vi "BuildPacket.vi"(1 "Data":u8[](array[numeric]), 2 "TxID":u32) -> (0 "MsgTX 2":T1)   [LabVIEW 2010]
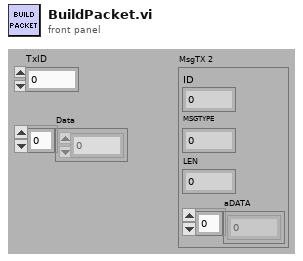
[diagram p1: front panel]
types:
  T1 = cluster{"ID":u32, "MSGTYPE":u8, "LEN":u8, "aDATA":u8[]}
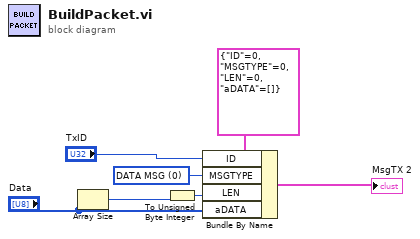
[diagram p0: block diagram]
diagram:
  w7 = u8 0 items=["STATUS"=128, "EXTENDED"=2, "RTR"=1, "DATA MSG"=0] ("MSGTYPE")
  n1 = Array Size(array="Data") -> (size(s)=w1:i32)
  n2 = To Unsigned Byte Integer(number=w1) -> (unsigned 8bit integer=w5:u8)
  n3 = Bundle By Name(cluster=T1 {"ID"=0, "MSGTYPE"=0, "LEN"=0, "aDATA"=[]} ("MsgTX 2"), "ID"="TxID", "MSGTYPE"=w7, "LEN"=w5, "aDATA"="Data") -> (→"MsgTX 2":T1)
